vi "nav4.vi"(9 "Drone":T3, 11 "Field":T1[][](array[typedef])) -> (2 "Move?":bool, 3 "direction":T2 items=["^", "^>", ">", "V>", "V", "<V", "<", "<^"])   [LabVIEW 2009]
uses:
  Drone data.ctl
  direction.ctl
  square.ctl
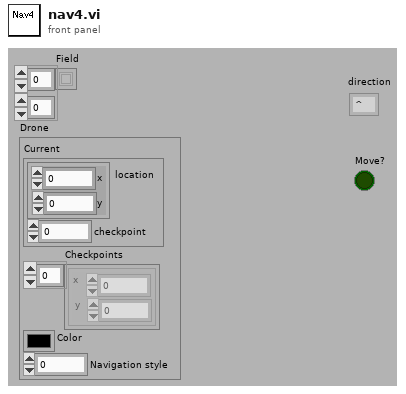
[diagram p1: front panel]
types:
  T1 = typedef "square.ctl" = u8
  T2 = typedef "direction.ctl" = i8
  T3 = typedef "Drone data.ctl" = cluster{"Current":cluster{"location":cluster{"x":i16, "y":i16}, "checkpoint":i32}, "Checkpoints":cluster{"x":i16, "y":i16}[], "Color":u32, "Navigation style":i32}
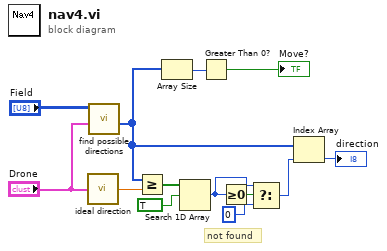
[diagram p0: block diagram]
diagram:
  # "not found"
  n1 = call "ideal direction.vi"("Drone"="Drone") -> ("ideal direction"=w8:dbl)
  n2 = call "find possible directions.vi"("Drone"="Drone", "Field"="Field") -> ("possible directions"=w7:T2[])  [unwired: 8 in, 1 out]
  n3 = Greater Or Equal?(x=w7, y=w8) -> (x >= y?=w6:bool[])
  n4 = Array Size(array=w7) -> (size(s)=w11:i32)
  n5 = Search 1D Array(1D array=w6, element=TRUE) -> (index of element=w3:i32)  [unwired: 1 in]
  n6 = Greater Than 0?(x=w11) -> (x > 0?=→"Move?":bool)
  n7 = Greater Or Equal To 0?(x=w3) -> (x >= 0?=w4:bool)
  n8 = Select(t=w3, s=w4, f=0) -> (s? t:f=w2:i32)
  n9 = Index Array(array=w7, index=w2) -> (element=→"direction":T2)
